vi "GetProperties.vi"(8 "error in":errorcluster, 11 "Numeric Text in":refnum<class "NumericText.lvclass">) -> (0 "error out":errorcluster, 3 "Numeric Text out":refnum<class "NumericText.lvclass">)   [LabVIEW 2014, in "NumericText.lvclass"]
uses:
  NumericText.lvclass
  NumericText.lvclass/NumericText.ctl
  Text/Text.lvclass
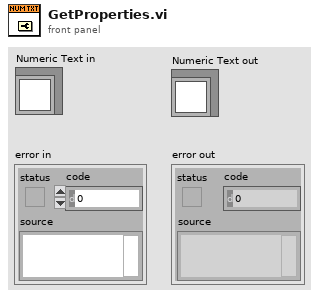
[diagram p1: front panel]
types:
  T1 = typedef "LVFormatAndPrecisionTypeDef.ctl" = cluster{"Format":u8, "Precision":u8}
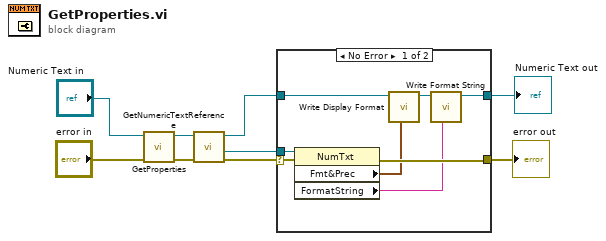
[diagram p0: block diagram]
diagram:
  n1 = call-parent "GetProperties.vi"("error in"="error in", "Text in"="Numeric Text in") -> ("error out"=w3:errorcluster, "Text out"=w4:refnum<class "NumericText.lvclass">)  [unwired: 8 in]
  n2 = call "GetNumericTextReference.vi"("error in"=w3, "Numeric Text in"=w4) -> ("error out"=w8:errorcluster, "NumericText reference"=w7:refnum<vi>, "Numeric Text out"=w6:refnum<class "NumericText.lvclass">)  [unwired: 7 in]
  n3 = case shown="No Error" w8 {
    selector: w8 -> [w17 w19]
    tunnel: [w15 w19] -> w9
    tunnel: w7 -> [w16 _]
    tunnel: w6 -> [w13 w18]
    tunnel: [w11 w18] -> w5
    frame No Error {
      n4 = property class="NumTxt"(reference=w16, error in=w17) -> (error out=w15:errorcluster, "Fmt&Prec"=w14:T1, "FormatString"=w10:string)  [unwired: 1 out]
      n5 = call "Write Display Format.vi"("Display Format"=w14, "NumericText in"=w13) -> ("NumericText out"=w12:refnum<class "NumericText.lvclass">)  [unwired: 7 in]
      n6 = call "Write Format String.vi"("Format String"=w10, "NumericText in"=w12) -> ("NumericText out"=w11:refnum<class "NumericText.lvclass">)  [unwired: 7 in]
    }
    frame Error {
    }
  }
  "error out" <- w9
  "Numeric Text out" <- w5
